vi "frequency_sweep_frequency_smooth.vi"(0 "Frequency":dbl[](array[numeric]), 1 "Channel (1:Channel 1)":i32, 2 "Amplitude (1.0 Vpp)":dbl=1.0 min=0.001 max=20.0 step=1.0 format="%#.3f", 3 "DC Offset (0.00 V)":dbl min=-10.0 max=10.0, 4 "SG Device 2":T1(ring) caption="Signal Generator Device", 5 "Modulation frequency":dbl, 6 "Current Sweep Value":refnum<vi>, 7 "Delay":dbl, 8 "Start t":refnum<vi>, 9 "Modulation Depth (0.0 %)":dbl, 11 "error in (no error)":errorcluster, 12 "Siglent Name":refnum<visa-resource-name>="USB0::0xF4EC::0x1102::SDG2XCAD4R3627::INSTR", 13 "AD2 2":i32, 14 "Stop 2":bool) -> (15 "error out":errorcluster)   [LabVIEW 2024, in "Sweep.lvlib"]
uses:
  Sweep.lvlib
  AD2/Node Parameters.ctl
  <instrlib>/Siglent SDG 1000 5000 800 Series/Public/Configure/Configure Modulation (AM).vi
  <instrlib>/Siglent SDG 1000 5000 800 Series/Siglent SDG 1000 5000 800 Series.lvlib
  AD2/AD2 DLL.lvlib
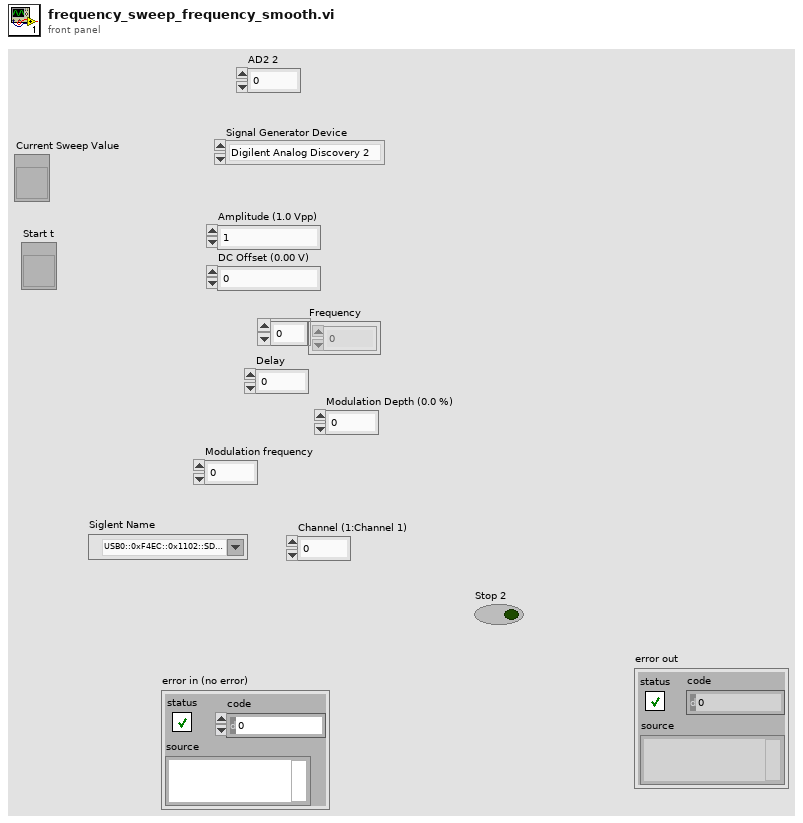
[diagram p1: front panel]
types:
  T1 = enum16{"Digilent Analog Discovery 2", "Siglent DG"}
  T2 = typedef "AD2 DLL.lvlib/Node Parameters.ctl" = cluster{"Function":u8, "Frequency":dbl, "Amplitude":dbl, "DC Offset":dbl, "Duty Cycle":dbl, "Phase":dbl}
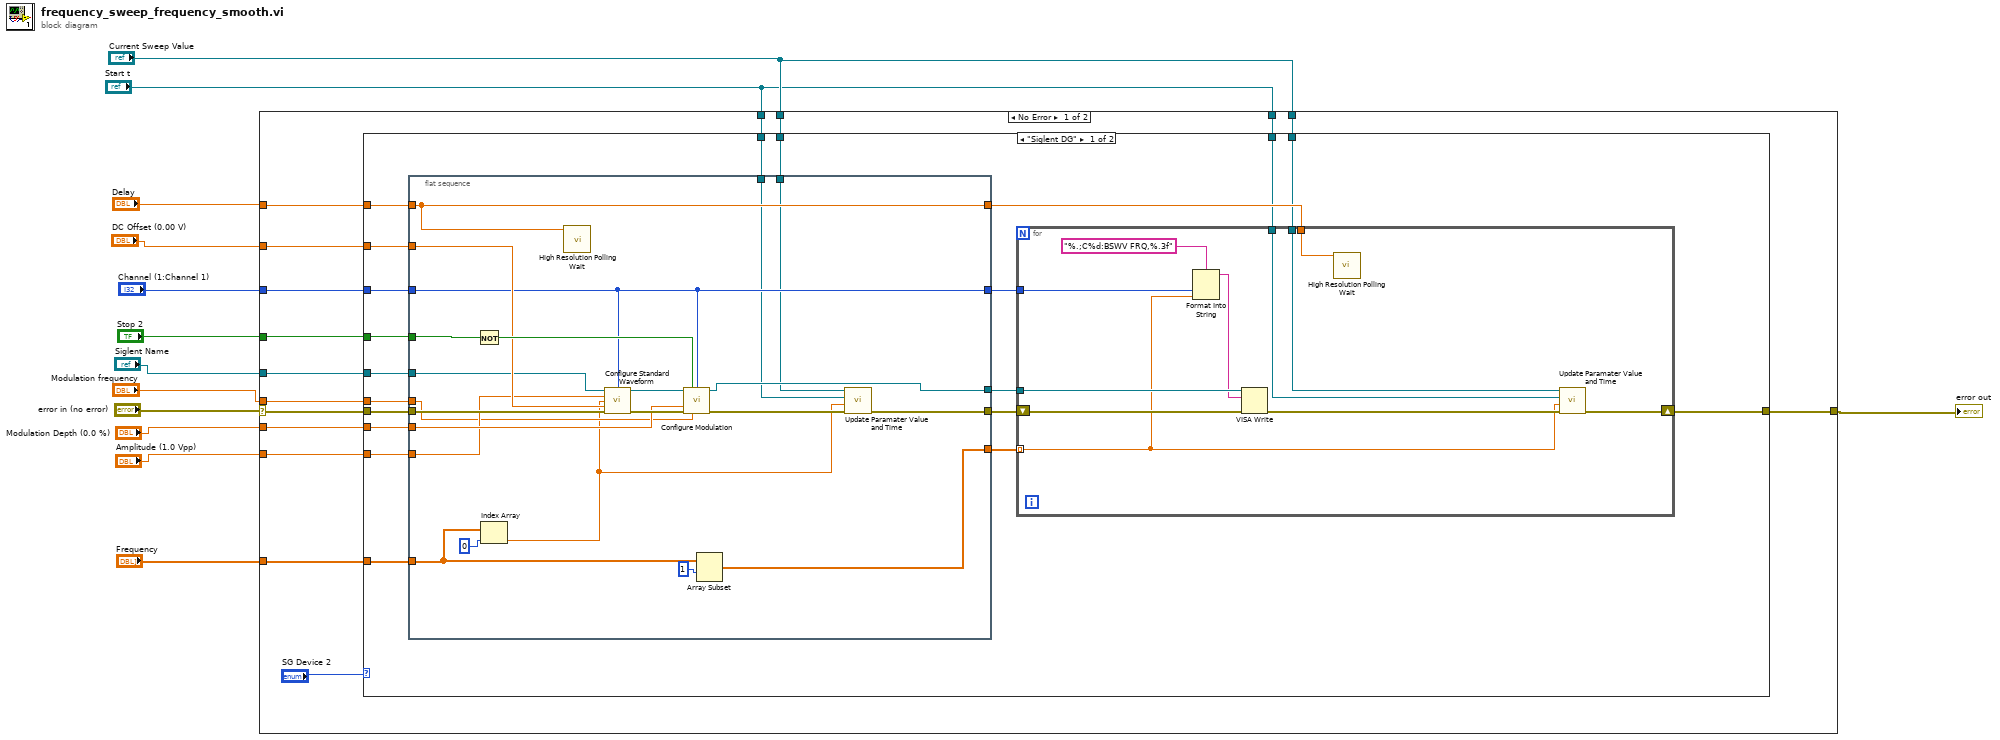
[diagram p0: block diagram]
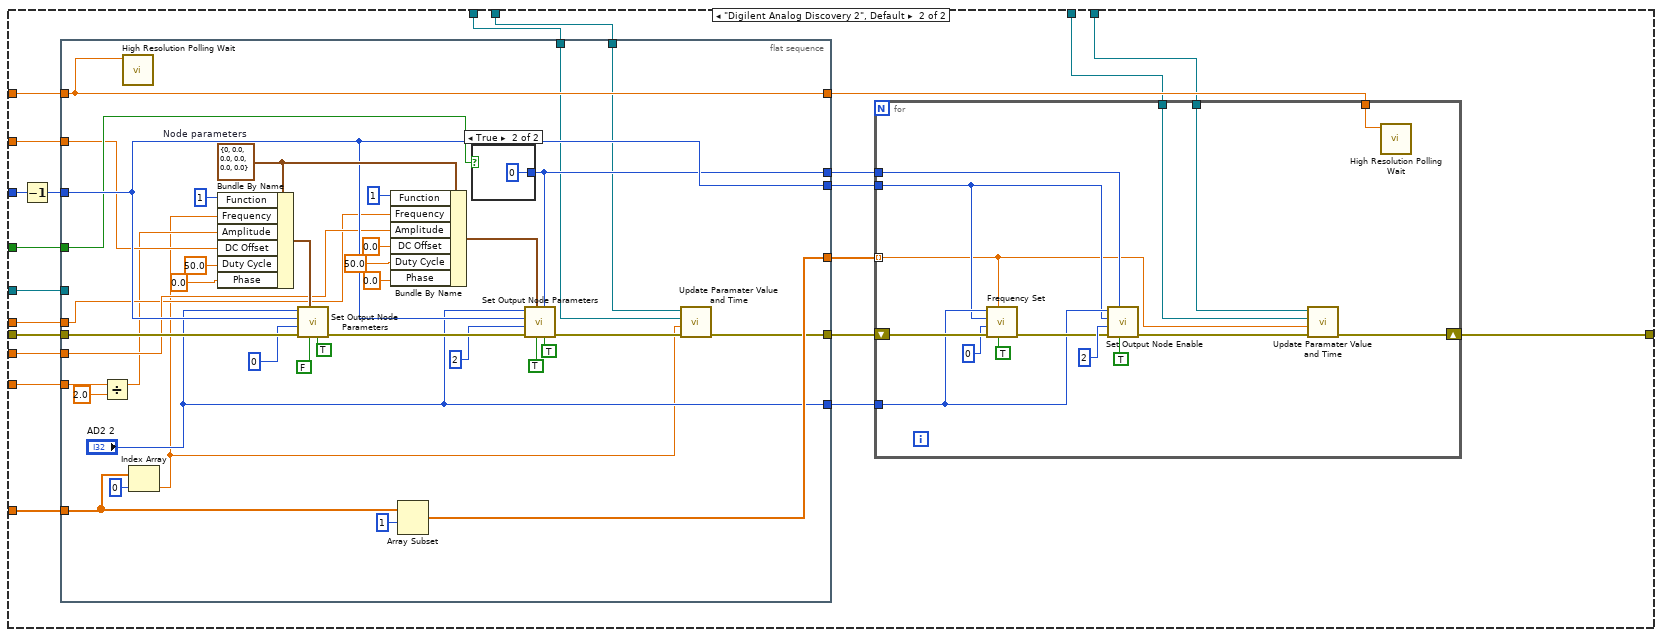
[diagram p2: hidden frame]
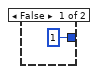
[diagram p3: hidden frame]
diagram:
  n1 = case shown="No Error" "error in (no error)" {
    selector: "error in (no error)" -> [w19 w160]
    tunnel: "Modulation Depth (0.0 %)" -> [w29 _]
    tunnel: "Amplitude (1.0 Vpp)" -> [w28 _]
    tunnel: "Modulation frequency" -> [w27 _]
    tunnel: "Stop 2" -> [w26 _]
    tunnel: [w25 w160] -> w12
    tunnel: "Frequency" -> [w24 _]
    tunnel: "Channel (1:Channel 1)" -> [w23 _]
    tunnel: "Delay" -> [w22 _]
    tunnel: "DC Offset (0.00 V)" -> [w21 _]
    tunnel: "Siglent Name" -> [w20 _]
    tunnel: "Current Sweep Value" -> [w17 _]
    tunnel: "Current Sweep Value" -> [w16 _]
    tunnel: "Start t" -> [w15 _]
    tunnel: "Start t" -> [w14 _]
    frame No Error {
      n2 = case shown="\"Siglent DG\"" "SG Device 2" {
        tunnel: w29 -> [w48 w104]
        tunnel: w28 -> [w47 w103]
        tunnel: w27 -> [w46 w102]
        tunnel: w26 -> [w45 w101]
        tunnel: [w43 w99] -> w25
        tunnel: w24 -> [w42 w98]
        tunnel: w23 -> [w40 w96]
        tunnel: w22 -> [w39 w95]
        tunnel: w21 -> [w38 w94]
        tunnel: w20 -> [w37 w93]
        tunnel: w19 -> [w36 w92]
        tunnel: w17 -> [w33 w86]
        tunnel: w16 -> [w32 w85]
        tunnel: w15 -> [w31 w84]
        tunnel: w14 -> [w30 w83]
        frame "Siglent DG" {
          n3 = flat-sequence {
            tunnel: [w70] -> w49
            tunnel: w48 -> [w67]
            tunnel: w47 -> [w56]
            tunnel: w46 -> [w55]
            tunnel: w45 -> [w66]
            tunnel: [w53] -> w44
            tunnel: w42 -> [w64]
            tunnel: [w62] -> w41
            tunnel: w40 -> [w57]
            tunnel: w39 -> [w58]
            tunnel: w38 -> [w61]
            tunnel: w37 -> [w60]
            tunnel: w36 -> [w59]
            tunnel: [w58] -> w35
            tunnel: [w57] -> w34
            tunnel: w33 -> [w52]
            tunnel: w31 -> [w51]
            frame #0 {
              n4 = Not(x=w66) -> (.not. x?=w71:bool)
              n5 = Index Array(array=w64, index=0) -> (element=w50:dbl)
              n6 = call <vilib>:"High Resolution Polling Wait.vi"("seconds to wait"=w58) -> ()  [unwired: 10 in, 1 out]
              n7 = call <instrlib>:"Configure Standard Waveform.vi"("VISA resource name"=w60, "Channel (1:Channel 1)"=w57, "Amplitude (1.0 Vpp)"=w56, "Frequency (1000 Hz)"=w50, "DC Offset (0.00 V)"=w61, "error in (no error)"=w59) -> ("VISA resource name out"=w68:refnum<visa-resource-name>, "error out"=w69:errorcluster)  [unwired: 8 in]
              n8 = call-poly <instrlib>:"Configure Modulation.vi"("VISA resource name"=w68, "Enable Amplitude Modulation (T:Enable)"=w71, "Channel (1:Channel 1)"=w57, "Modulation Depth (0.0 %)"=w67, "error in (no error)"=w69, "Modulation Frequency (100 Hz)"=w55) -> ("VISA resource name out"=w70:refnum<visa-resource-name>, "error out"=w54:errorcluster)  [unwired: 8 in]
              n9 = Array Subset "Array Subset"(array=w64, index=1) -> (w62:dbl[])  [unwired: 1 in]
              n10 = call "Update Paramater Value and Time.vi"("error in (no error)"=w54, "Value"=w50, "Start t"=w51, "Current Sweep Value"=w52) -> ("error out"=w53:errorcluster)  [unwired: 7 in]
            }
          }
          n11 = for {
            shift-right: [w75] -> w43
            shift-left: w44 -> [w78]
            tunnel: w49 -> [w80]
            tunnel: w35 -> [w77]
            tunnel: w41 -> [w72] mode=indexing
            tunnel: w34 -> [w82]
            tunnel: w32 -> [w74]
            tunnel: w30 -> [w73]
            n12 = Format Into String(format string="%.;C%d:BSWV FRQ,%.3f", w82, w72) -> (resulting string=w79:string)  [unwired: 2 in, 1 out]
            n13 = VISA Write(VISA resource name=w80, write buffer=w79, error in (no error)=w78) -> (error out=w76:errorcluster)  [unwired: 2 out]
            n14 = call <vilib>:"High Resolution Polling Wait.vi"("seconds to wait"=w77) -> ()  [unwired: 10 in, 1 out]
            n15 = call "Update Paramater Value and Time.vi"("error in (no error)"=w76, "Value"=w72, "Start t"=w73, "Current Sweep Value"=w74) -> ("error out"=w75:errorcluster)  [unwired: 7 in]
          }
        }
        frame "Digilent Analog Discovery 2", Default {
          n16 = Decrement(x=w96) -> (x-1=w90:i32)
          n17 = flat-sequence {
            tunnel: w104 -> [w120]
            tunnel: w103 -> [w113]
            tunnel: w102 -> [w112]
            tunnel: w101 -> [w121]
            tunnel: [w108] -> w100
            tunnel: w98 -> [w141]
            tunnel: [w139] -> w97
            tunnel: w90 -> [w124]
            tunnel: w95 -> [w138]
            tunnel: w94 -> [w116]
            tunnel: w93 -> [_]
            tunnel: w92 -> [w137]
            tunnel: [w138] -> w87
            tunnel: [w124] -> w91
            tunnel: ["AD2 2"] -> w89
            tunnel: [w115] -> w88
            tunnel: w86 -> [w106]
            tunnel: w84 -> [w105]
            frame #0 {
              w128 = T2 {"Function"=0, "Frequency"=0.0, "Amplitude"=0.0, "DC Offset"=0.0, "Duty Cycle"=0.0, "Phase"=0.0}  # Node parameters
              n18 = Divide(x=w113, y=2.0) -> (x/y=w111:dbl)
              n19 = call <vilib>:"High Resolution Polling Wait.vi"("seconds to wait"=w138) -> ()  [unwired: 10 in, 1 out]
              n20 = Index Array(array=w141, index=0) -> (element=w107:dbl)
              n21 = Bundle By Name(cluster=w128, "Function"=u8 1, "Frequency"=w107, "Amplitude"=w111, "DC Offset"=w116, "Duty Cycle"=50.0, "Phase"=0.0) -> (w135:T2)
              n22 = call "Set Output Node Parameters.vi"("Apply parameters"=TRUE, "Use Enable"=FALSE, "Node parameters"=w135, "error in (no error)"=w137, "node"=0, "idxChannel"=w124, "hdwf"="AD2 2") -> ("error out"=w136:errorcluster)  [unwired: 3 in, 1 out]
              n23 = Bundle By Name(cluster=w128, "Function"=u8 1, "Frequency"=w112, "Amplitude"=w120, "DC Offset"=0.0, "Duty Cycle"=50.0, "Phase"=0.0) -> (w127:T2)
              n24 = Array Subset "Array Subset"(array=w141, index=1) -> (w139:dbl[])  [unwired: 1 in]
              n25 = case shown="True" w121 {
                tunnel: [1 ("Enable") 0 ("Enable")] -> w115
                frame False {
                }
                frame True {
                }
              }
              n26 = call "Set Output Node Parameters.vi"("Apply parameters"=TRUE, "Enable"=w115, "Use Enable"=TRUE, "Node parameters"=w127, "error in (no error)"=w136, "node"=2, "idxChannel"=w124, "hdwf"="AD2 2") -> ("error out"=w109:errorcluster)  [unwired: 2 in, 1 out]
              n27 = call "Update Paramater Value and Time.vi"("error in (no error)"=w109, "Value"=w107, "Start t"=w105, "Current Sweep Value"=w106) -> ("error out"=w108:errorcluster)  [unwired: 7 in]
            }
          }
          n28 = for {
            shift-right: [w148] -> w99
            shift-left: w100 -> [w155]
            tunnel: w97 -> [w146] mode=indexing
            tunnel: w91 -> [w152]
            tunnel: w89 -> [w153]
            tunnel: w88 -> [w158]
            tunnel: w87 -> [w157]
            tunnel: w85 -> [w147]
            tunnel: w83 -> [w145]
            n29 = call "Frequency Set.vi"("Update"=TRUE, "Frequency"=w146, "error in (no error)"=w155, "node"=0, "idxChannel"=w152, "hdwf"=w153) -> ("error out"=w154:errorcluster)  [unwired: 3 in, 2 out]
            n30 = call "Set Output Node Enable.vi"("Update"=TRUE, "Enable"=w158, "error in (no error)"=w154, "node"=2, "idxChannel"=w152, "hdwf"=w153) -> ("error out"=w149:errorcluster)  [unwired: 4 in, 1 out]
            n31 = call "Update Paramater Value and Time.vi"("error in (no error)"=w149, "Value"=w146, "Start t"=w145, "Current Sweep Value"=w147) -> ("error out"=w148:errorcluster)  [unwired: 7 in]
            n32 = call <vilib>:"High Resolution Polling Wait.vi"("seconds to wait"=w157) -> ()  [unwired: 10 in, 1 out]
          }
        }
      }
    }
    frame Error {
    }
  }
  "error out" <- w12
